vi "Update Serial Stream.vi"(7 "Device Number":T1, 11 "Stream Type":T2) -> ()   [LabVIEW 2016]
uses:
  TypeDefs/Z900_navX_ActionTypeDef.ctl
  navX Library v2.lvlib
  TypeDefs/Z900_navX_SerialStreamTypeDef.ctl
  TypeDefs/FRIC_navX_DeviceNumbersTypeDef.ctl
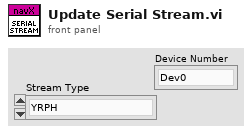
[diagram p1: front panel]
types:
  T1 = typedef "FRIC_navX_DeviceNumbersTypeDef.ctl" = enum16{"Dev0", "Dev1", "Dev2", "Dev3"}
  T2 = typedef "navX Library v2.lvlib/Z900_navX_SerialStreamTypeDef.ctl" = enum16{"YRPH", "Quaterinons", "Gyro/Raw", "AHRS", "AHRSAndPositioning"}
  T3 = typedef "navX Library v2.lvlib/Z900_navX_ActionTypeDef.ctl" = enum16{"None", "Halt", "Update Serial Protocol", "Zero-Yaw", "Zero-Displacement", "Zero-Velocity"}
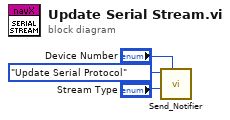
[diagram p0: block diagram]
diagram:
  n1 = call "Send_Notifier.vi"("Device Number"="Device Number", "Stream Type"="Stream Type", "navX Action"=Z900_navX_ActionTypeDef."Update Serial Protocol") -> ()  [unwired: 9 in]
